vi "ex1_snap Color.vi"() -> ()   [LabVIEW 2012]
panel:
  in  "Blue Exposure":u32=100000
  in  "Red Exposure":u32=100000
  in  "Green Exposure":u32=100000
  out "error status":errorcluster
  out "Preview Window":picture
  # "usec"
  # "usec"
  # "usec"
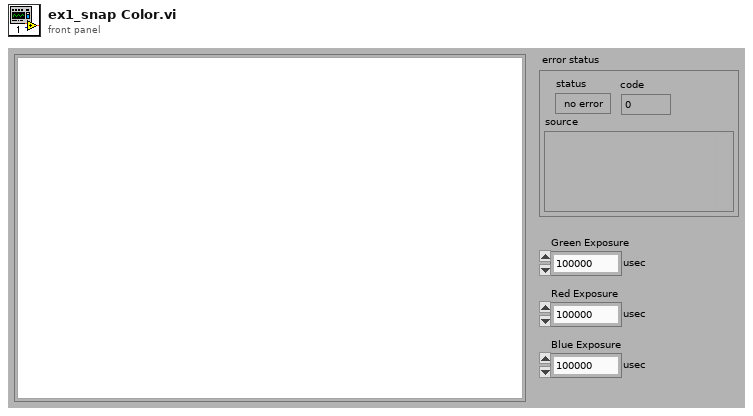
[diagram p1: front panel]
types:
  T1 = typedef "Image Type" = u32
  T2 = cluster{"Green Exposure":u32, "Red Exposure":u32, "Blue Exposure":u32}
  T3 = typedef "IMAQ Image.ctl" = refnum<image>
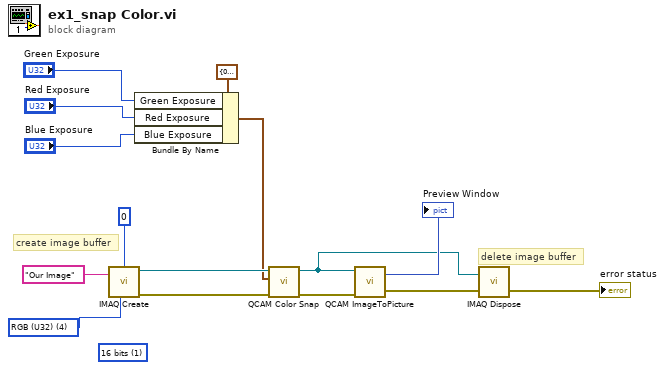
[diagram p0: block diagram]
diagram:
  w1 = T1 4 items=["Grayscale (U8)", "Grayscale (I16)", "Grayscale (SGL)", "Complex (CSG)", "RGB (U32)", "HSL (U32)", "RGB (U64)"] ("Image Type")
  (unwired) u32 1 items=["8 bits", "16 bits"] ("Image Type")
  # "create image buffer"
  # "delete image buffer"
  n1 = call "IMAQ Create"("Border Size"=0, "Image Name"="Our Image", "Image Type"=w1) -> ("New Image"=w14:T3, "error out"=w11:errorcluster)  [unwired: 1 in, 1 out]
  n2 = Bundle By Name(cluster=T2 {"Green Exposure"=0, "Red Exposure"=0, "Blue Exposure"=0} ("Exposures"), "Green Exposure"="Green Exposure", "Red Exposure"="Red Exposure", "Blue Exposure"="Blue Exposure") -> (w2:T2)
  n3 = call <userlib>:"QCAM Color Snap.vi"("error in (no error)"=w11, "Exposures"=w2, "New Image"=w14) -> ("error out"=w12:errorcluster, "Image Out"=w9:T3)  [unwired: 2 in, 5 out]
  n4 = call <userlib>:"QCAM ImageToPicture.vi"("error in (no error)"=w12, "Image"=w9) -> ("error out"=w13:errorcluster, "Picture Out"=→"Preview Window":picture)
  n5 = call "IMAQ Dispose"("Image"=w9, "error in (no error)"=w13) -> ("error out"=→"error status":errorcluster)  [unwired: 1 in, 3 out]
